vi "integrated data gatherer.vi"(0 "tdms file":refnum<k34>, 1 "time stamp":timestamp, 2 "lockin information":T1, 3 "lvdt":cluster{dbl, dbl, dbl, dbl, dbl, dbl}, 4 "v0":dbl[](array[numeric]) format="%#_6p", 5 "v1":dbl[](array[numeric]) format="%#_6p", 6 "data":dbl[](array[numeric]), 7 "tip voltage":dbl) -> (10 "TtG":dbl, 11 "FtG":dbl, 12 "TtR":dbl, 13 "FtR":dbl, 14 "tdms file out":refnum<k34>, 15 "z":dbl, 16 "x":dbl, 17 "y":dbl, 18 "deflection":dbl format="%#_13g", 19 "vt":dbl)   [LabVIEW 2013]
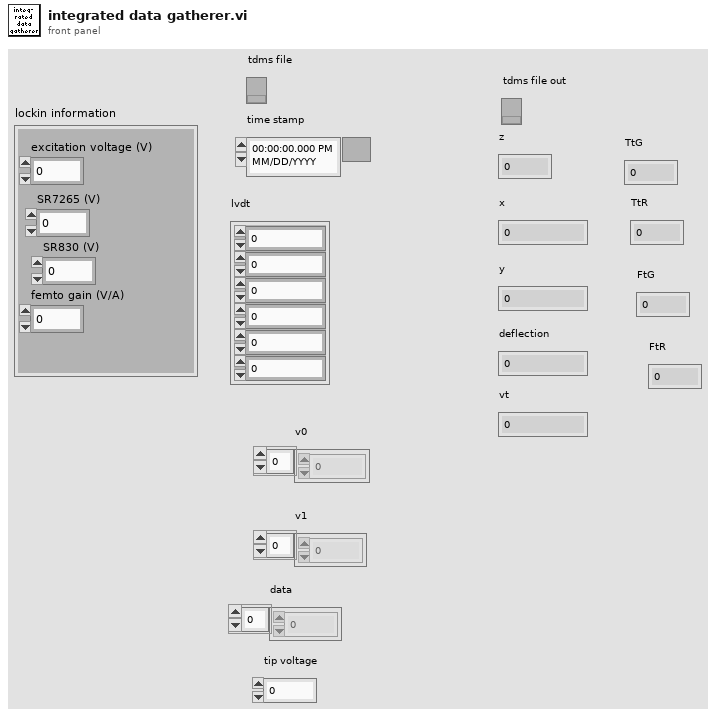
[diagram p1: front panel]
types:
  T1 = cluster{"excitation voltage (V)":dbl, "SR7265 (V)":dbl, "SR830 (V)":dbl, "femto gain (V/A)":dbl}
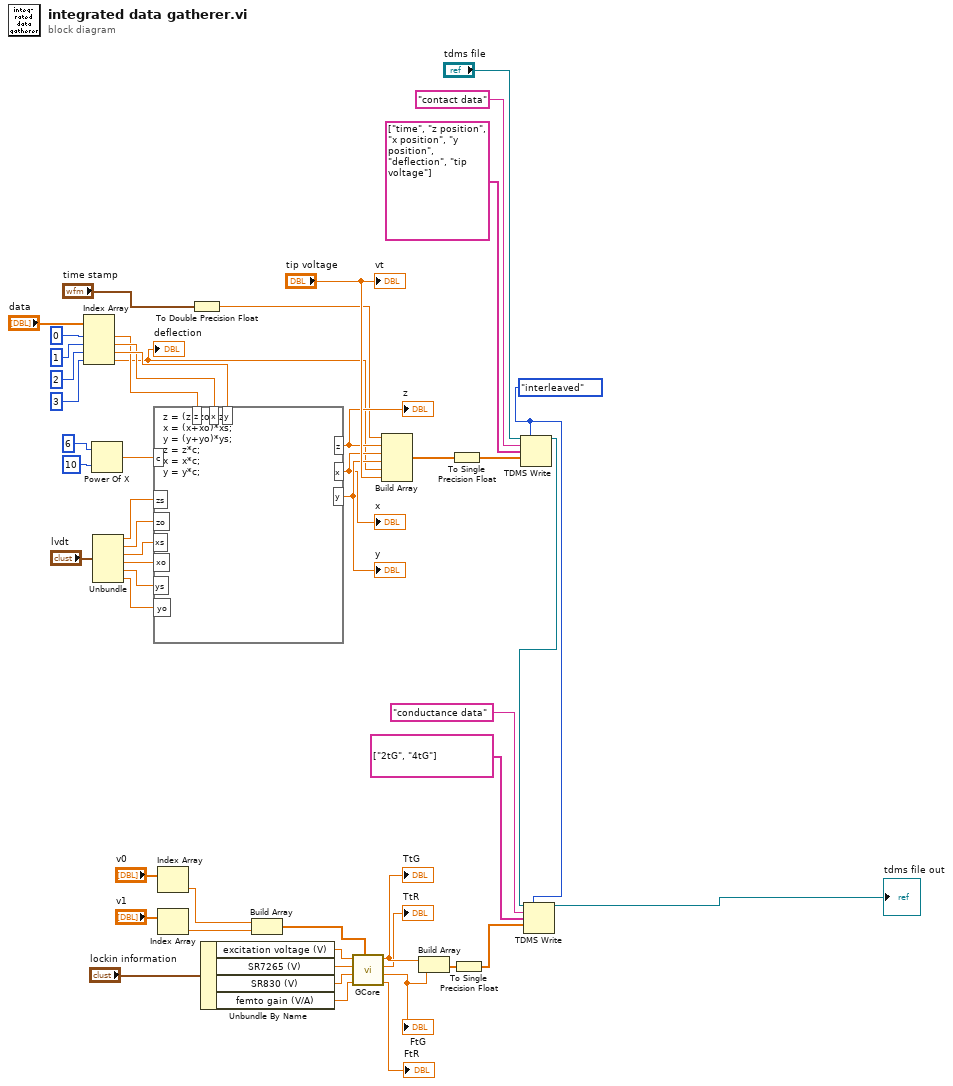
[diagram p0: block diagram]
diagram:
  w1 = enum16{"decimated", "interleaved"}."interleaved" ("data layout (0:decimated)")
  n1 = Index Array(array="data", index #1=0, index #2=1, index #3=2, index #4=3) -> (element #1=w34:dbl, element #2=w35:dbl, element #3=w36:dbl, element #4=w28:dbl)
  "deflection" <- w28
  n2 = Power Of X(1:10, 2:6) -> (0:w47:dbl)
  n3 = Unbundle("lvdt") -> (w39:dbl, w40:dbl, w41:dbl, w42:dbl, w43:dbl, w44:dbl)
  n4 = formula code="z = (z+zo)*zs;\nx = (x+xo)*xs;\ny = (y+yo)*ys;\nz = z*c;\nx = x*c;\ny = y*c;"("z"=w34, "x"=w35, "y"=w36, "zo"=w40, "xs"=w41, "xo"=w42, "ys"=w43, "zs"=w39, "yo"=w44, "c"=w47) -> ("z"=w48:dbl, "x"=w49:dbl, "y"=w50:dbl)
  "y" <- w50
  "x" <- w49
  "z" <- w48
  n5 = Index Array(array="v0") -> (element=w9:dbl)  [unwired: 1 in]
  n6 = Index Array(array="v1") -> (element=w7:dbl)  [unwired: 1 in]
  n7 = To Double Precision Float(number="time stamp") -> (double precision float=w37:dbl)
  n8 = Unbundle By Name("lockin information") -> ("excitation voltage (V)"=w15:dbl, "SR7265 (V)"=w14:dbl, "SR830 (V)"=w13:dbl, "femto gain (V/A)"=w12:dbl)
  n9 = Build Array(w9, w7) -> (w17:dbl[])
  n10 = call "GCore.vi"("G data"=w17, "Femto Gain (V/A)"=w12, "SR830 sensitivity"=w13, "SR7265 sensitivity (V)"=w14, "Excitation voltage (V)"=w15) -> ("4tR"=→"FtR":dbl, "4tG"=w6:dbl, "2tR"=→"TtR":dbl, "2tG"=w11:dbl)
  "TtG" <- w11
  "FtG" <- w6
  n11 = Build Array(w37, w48, w49, w50, w28, "tip voltage") -> (w25:dbl[])
  n12 = Build Array(w11, w6) -> (w21:dbl[])
  n13 = To Single Precision Float(number=w25) -> (single precision float=w24:sgl[])
  n14 = To Single Precision Float(number=w21) -> (single precision float=w20:sgl[])
  n15 = TDMS Write(0:"tdms file", 1:w1, 5:"contact data", 7:string[] ["time", "z position", "x position", "y position", "deflection", "tip voltage"], 9:w24) -> (4:w3:refnum<k34>)  [unwired: 1 in, 3 out]
  n16 = TDMS Write(0:w3, 1:w1, 5:"conductance data", 7:string[] ["2tG", "4tG"], 9:w20) -> (4:→"tdms file out":refnum<k34>)  [unwired: 1 in, 3 out]
  "vt" <- "tip voltage"
